vi "Test Publish QoS 0 Latency.vi"() -> ()   [LabVIEW 2013]
uses:
  <vilib>/LabVIEW Open Source Project/MQTT Control Packets/Control Packets/ControlPacket/Control Packet Type -- enum.ctl
  <vilib>/LabVIEW Open Source Project/MQTT Control Packets/Control Packets/ControlPacket/ControlPacket.lvclass
  <vilib>/LabVIEW Open Source Project/MQTT Control Packets/Control Packets/ControlPacket/QualityOfService -- enum.ctl
  <vilib>/LabVIEW Open Source Project/MQTT Control Packets/Control Packets/PUBLISH/PUBLISH.lvclass
  <vilib>/LabVIEW Open Source Project/MQTT Control Packets/Control Packets/ControlPacket/ControlPacket.lvclass/ControlPacket.ctl
  source/Client class/Client.lvclass
  <vilib>/LabVIEW Open Source Project/MQTT Connection/MQTT_Base/Base Class/MQTT_Base.lvclass
  <vilib>/LabVIEW Open Source Project/MQTT Control Packets/Control Packets/CONNACK/CONNACK.lvclass
  <vilib>/LabVIEW Open Source Project/Connection/Connection.TCP/Connection.TCP.lvclass
  <vilib>/LabVIEW Open Source Project/Connection/Connection/Connection.lvclass
panel:
  out "Raw Reception Latency (s)":dbl
  out "bytes received":i32
  out "Waveform Chart":cluster{dbl, dbl}(graph)
  out "# Bytes in payload":i32[](array[numeric])
  out "Disconnected by peer":bool
  out "# packets received":i32
  out "Raw Publication Latency (s)":dbl
  out "Topic":string[](array[string])
  out "Packet Type":T1[](array[typedef])
  out "server connected":bool
  out "listener error":errorcluster
  out "error out":errorcluster
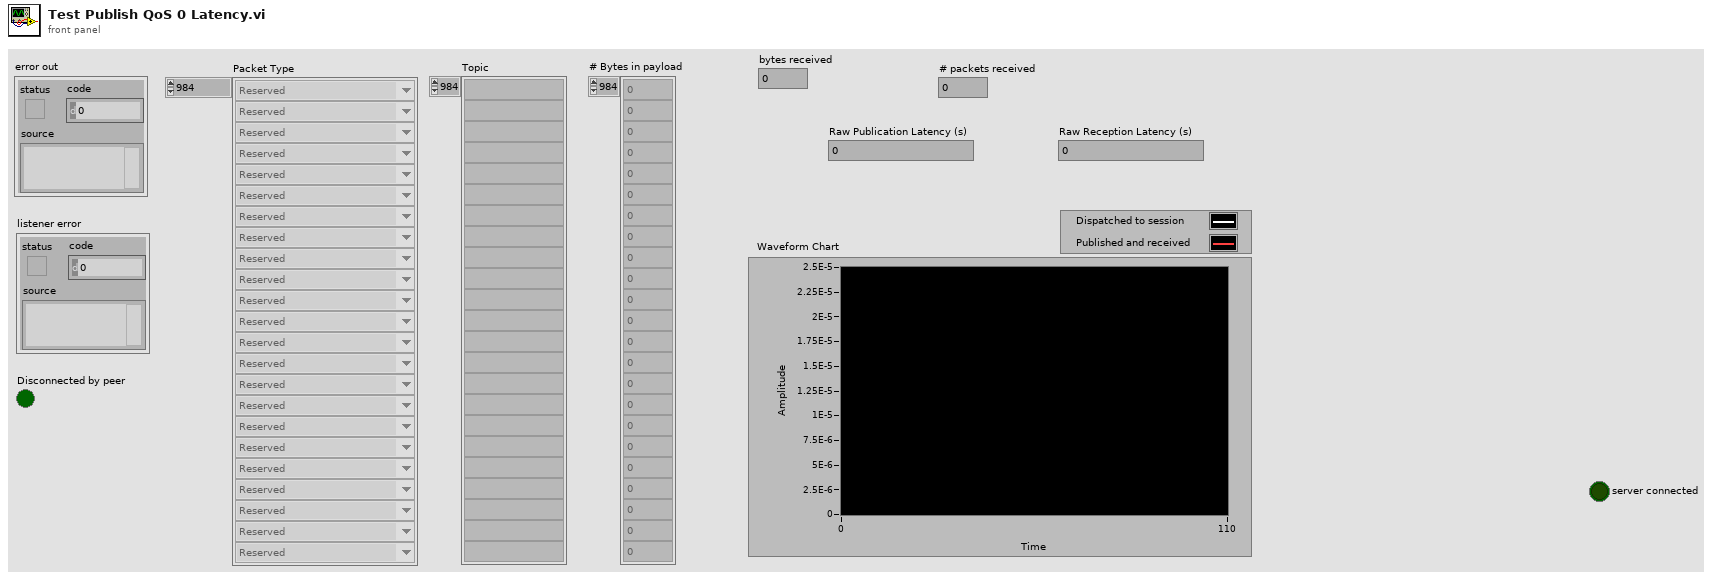
[diagram p1: front panel]
types:
  T1 = typedef "MQTT_Control_Packets.lvlib/ControlPacket.lvclass/Control Packet Type -- enum.ctl" = enum16{"Reserved", "CONNECT", "CONNACK", "PUBLISH", "PUBACK", "PUBREC", "PUBREL", "PUBCOMP", "SUBSCRIBE", "SUBACK", "UNSUBSCRIBE", "UNSUBACK", "PINGREQ", "PINGRESP", "DISCONNECT", "AUTH"}
  T2 = enum16{"Standard", "Buffered", "CRLF", "Immediate"}
  T3 = typedef "MQTT_Control_Packets.lvlib/ControlPacket.lvclass/QualityOfService -- enum.ctl" = enum16{"0 (At Most Once)", "1 (At Least Once)", "2 (Exactly Once)"}
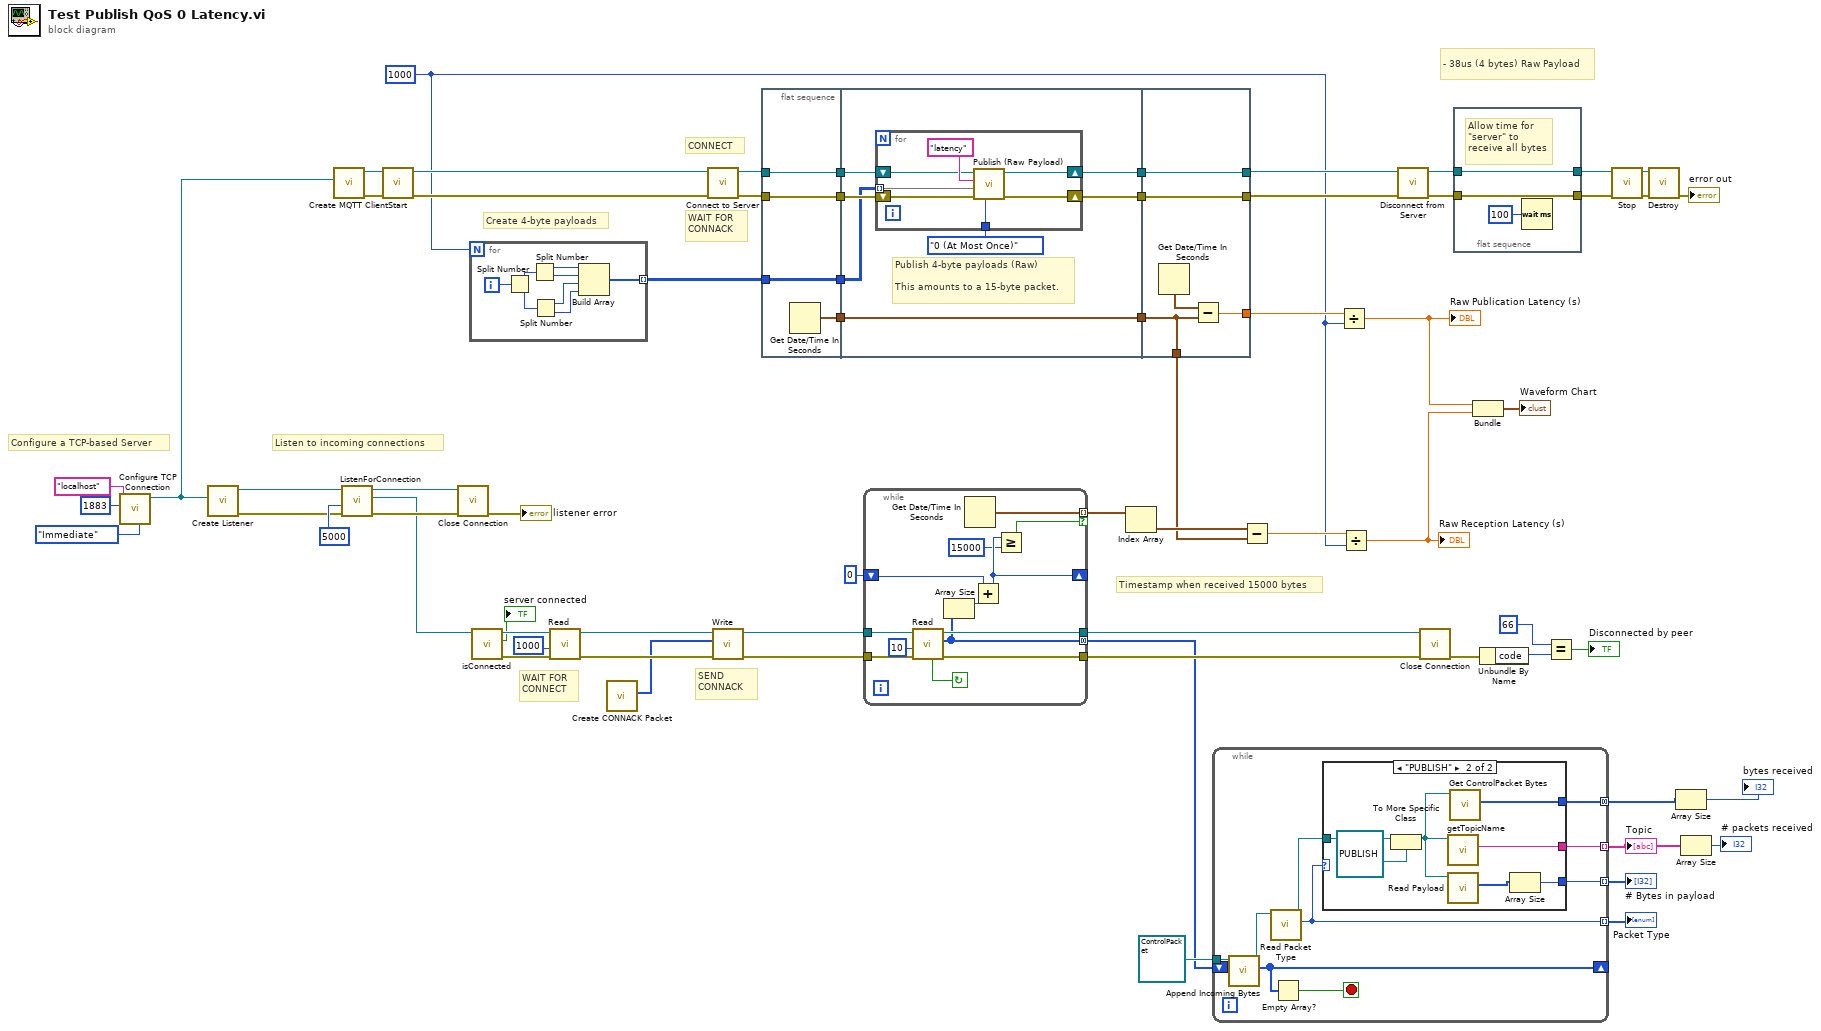
[diagram p0: block diagram]
diagram:
  w9 = 1000
  # "CONNECT"
  # "WAIT FOR\nCONNACK"
  # "Timestamp when received 15000 bytes"
  # "SEND \nCONNACK"
  # "WAIT FOR\nCONNECT"
  # "- 38us (4 bytes) Raw Payload"
  # "Create 4-byte payloads"
  # "Listen to incoming connections"
  # "Configure a TCP-based Server"
  n1 = call <vilib>:"Configure TCP Connection.vi"("Read Mode (Immediate)"=T2."Immediate", "remote port (80)"=u16 1883, "address (localhost)"="localhost") -> ("Connection.TCP"=w3:refnum<class "Connection.TCP.lvclass">)  [unwired: 7 in, 1 out]
  n2 = call <vilib>:"Create Listener.vi"("Connection Configuration"=w3) -> ("error out"=w2:errorcluster, "Listener"=w1:refnum<class "Connection.TCP.lvclass">)  [unwired: 9 in]
  n3 = call "Create MQTT Client.vi"("Connection Configuration"=w3) -> ("error out"=w66:errorcluster, "Client out"=w64:refnum<class "Client.lvclass">)  [unwired: 9 in]
  n4 = call <vilib>:"ListenForConnection.vi"("error in (no error)"=w2, "timeout (2000 ms)"=5000 ("bytes to read (100)"), "Listener"=w1) -> ("error out"=w59:errorcluster, "Connection"=w54:refnum<class "Connection.lvclass">, "Listener out"=w60:refnum<class "Connection.TCP.lvclass">)  [unwired: 5 in, 1 out]
  n5 = call <vilib>:"Start.vi"("error in (no error)"=w66, "MQTT_Base in"=w64) -> ("error out"=w65:errorcluster, "MQTT_Base out"=w63:refnum<class "Client.lvclass">)  [unwired: 7 in, 1 out]
  n6 = call <vilib>:"Close Connection.vi"("error in (no error)"=w59, "Connection in"=w60) -> ("error out"=→"listener error":errorcluster)  [unwired: 8 in, 1 out]
  n7 = for {
    N: w9 -> [_]
    tunnel: [w68] -> w44 mode=indexing
    i -> [w75]
    n8 = Split Number(x=w75) -> (hi(x)=w74:u16, lo(x)=w73:u16)
    n9 = Split Number(x=w74) -> (hi(x)=w72:u8, lo(x)=w71:u8)
    n10 = Split Number(x=w73) -> (hi(x)=w70:u8, lo(x)=w69:u8)
    n11 = Build Array(w72, w71, w70, w69) -> (w68:u8[])
  }
  n12 = call <vilib>:"isConnected.vi"("Connection in"=w54) -> ("error out"=w32:errorcluster, "connected"=→"server connected":bool, "Connection out"=w33:refnum<class "Connection.lvclass">)  [unwired: 8 in]
  n13 = call <vilib>:"Read.vi"("error in (no error)"=w32, "timeout (2000 ms)"=1000 ("bytes to read (100)"), "TCPConnection in"=w33) -> ("error out"=w34:errorcluster, "TCPConnection out"=w35:refnum<class "Connection.lvclass">)  [unwired: 4 in, 3 out]
  n14 = call <vilib>:"Create CONNACK Packet.vi"() -> ("Bytes Stream"=w30:u8[])  [unwired: 9 in, 2 out]
  n15 = call "Connect to Server.vi"("error in (no error)"=w65, "Client in"=w63) -> ("error out"=w53:errorcluster, "Client out"=w51:refnum<class "Client.lvclass">)  [unwired: 6 in, 2 out]
  n16 = call <vilib>:"Write.vi"("error in (no error)"=w34, "Bytes"=w30, "Connection in"=w35) -> ("error out"=w28:errorcluster, "Connection"=w29:refnum<class "Connection.lvclass">)  [unwired: 7 in]
  n17 = flat-sequence {
    tunnel: w51 -> [w78]
    tunnel: w53 -> [w79]
    tunnel: [w79] -> w49
    tunnel: [w78] -> w48
    tunnel: [w77] -> w45
    tunnel: w44 -> [w77]
    tunnel: [w76] -> w43
    tunnel: w49 -> [w86]
    tunnel: w48 -> [w84]
    tunnel: [w85] -> w47
    tunnel: [w83] -> w46
    tunnel: w45 -> [w82]
    tunnel: w43 -> [w80]
    tunnel: [w80] -> w42
    tunnel: [w97] -> w50
    tunnel: [w98] -> w52
    tunnel: w47 -> [w98]
    tunnel: w46 -> [w97]
    tunnel: w42 -> [w94]
    tunnel: [w95] -> w41
    tunnel: [w94] -> w5
    frame #0 {
      n18 = Get Date/Time In Seconds() -> (seconds since 1Jan1904=w76:timestamp)
    }
    frame #1 {
      # "Publish 4-byte payloads (Raw)\n\nThis amounts to a 15-byte packet."
      n19 = for {
        shift-right: [w91] -> w85
        shift-left: w86 -> [w90]
        shift-right: [w89] -> w83
        shift-left: w84 -> [w92]
        tunnel: w82 -> [w88] mode=indexing
        tunnel: QualityOfService_--_enum."0 (At Most Once)" ("QoS") -> [w87]
        n20 = call "Publish (Raw Payload).vi"("QoS"=w87, "error in (no error)"=w90, "Binary Payload"=w88, "Topic Name"="latency", "Client in"=w92) -> ("error out"=w91:errorcluster, "Client out"=w89:refnum<class "Client.lvclass">)  [unwired: 4 in, 1 out]
      }
    }
    frame #2 {
      n21 = Get Date/Time In Seconds() -> (seconds since 1Jan1904=w96:timestamp)
      n22 = Subtract(x=w96, y=w94) -> (x-y=w95:dbl)
    }
  }
  n23 = while {
    tunnel: w29 -> [w110]
    tunnel: w28 -> [w109]
    tunnel: [w108] -> w27
    tunnel: [w107] -> w26
    tunnel: [w105] -> w16 mode=concatenating
    shift-right: [w102] -> _
    shift-left: 0 ("size(s)") -> [w103]
    tunnel: [w100] -> w12 mode=indexing if=w99
    stop <- w106 continue-if-true
    n24 = call <vilib>:"Read.vi"("error in (no error)"=w109, "timeout (2000 ms)"=10 ("bytes to read (100)"), "TCPConnection in"=w110) -> ("error out"=w107:errorcluster, "Bytes"=w105:u8[], "TCPConnection out"=w108:refnum<class "Connection.lvclass">, "connected"=w106:bool)  [unwired: 4 in, 1 out]
    n25 = Array Size(array=w105) -> (size(s)=w104:i32)
    n26 = Get Date/Time In Seconds() -> (seconds since 1Jan1904=w100:timestamp)
    n27 = Add(x=w103, y=w104) -> (x+y=w102:i32)
    n28 = Greater Or Equal?(x=w102, y=15000) -> (x >= y?=w99:bool)
  }
  n29 = Index Array(array=w12) -> (element=w11:timestamp)  [unwired: 1 in]
  n30 = while {
    tunnel: refnum<class "ControlPacket.lvclass"> refnum ("Incomplete ControlPacket") -> [w120]
    shift-right: [w119] -> _
    shift-left: w16 -> [w121]
    tunnel: [w116] -> w24 mode=indexing
    tunnel: [w114] -> w23 mode=indexing
    tunnel: [w113] -> w17 mode=indexing
    tunnel: [w112] -> w15 mode=concatenating
    stop <- w118 stop-if-true
    n31 = call <vilib>:"Append Incoming Bytes.vi"("Incoming Packets"=w121, "Incomplete ControlPacket"=w120) -> ("Remaining Packets"=w119:u8[], "ControlPacket"=w117:refnum<class "ControlPacket.lvclass">)  [unwired: 6 in, 2 out]
    n32 = call <vilib>:"Read Packet Type.vi"("ControlPacket in"=w117) -> ("Control Packet Type"=w116:T1, "ControlPacket out"=w115:refnum<class "ControlPacket.lvclass">)  [unwired: 9 in]
    n33 = Empty Array?(array=w119) -> (empty?=w118:bool)
    n34 = case shown="\"PUBLISH\"" w116 {
      tunnel: w115 -> [_ w128]
      tunnel: [_ w126] -> w114
      tunnel: [_ w124] -> w113
      tunnel: [_ w122] -> w112
      frame Default {
      }
      frame "PUBLISH" {
        n35 = To More Specific Class(target class=refnum<class "PUBLISH.lvclass"> refnum ("PUBLISH in"), reference=w128) -> (specific class reference=w123:refnum<class "PUBLISH.lvclass">)  [unwired: 1 in, 1 out]
        n36 = call <vilib>:"getTopicName.vi"("PUBLISH in"=w123) -> ("Topic"=w126:string)  [unwired: 8 in, 2 out]
        n37 = call <vilib>:"Read Payload.vi"("ControlPacket in"=w123) -> ("Payload"=w125:u8[])  [unwired: 9 in, 1 out]
        n38 = call <vilib>:"Get ControlPacket Bytes.vi"("ControlPacket"=w123) -> ("Bytes Stream"=w122:u8[])  [unwired: 7 in, 3 out]
        n39 = Array Size(array=w125) -> (size(s)=w124:i32)
      }
    }
  }
  "Packet Type" <- w24
  "Topic" <- w23
  "# Bytes in payload" <- w17
  n40 = Subtract(x=w11, y=w5) -> (x-y=w10:dbl)
  n41 = Divide(x=w41, y=w9) -> (x/y=w7:dbl)
  "Raw Publication Latency (s)" <- w7
  n42 = Divide(x=w10, y=w9) -> (x/y=w8:dbl)
  "Raw Reception Latency (s)" <- w8
  n43 = call "Disconnect from Server.vi"("error in (no error)"=w52, "Client in"=w50) -> ("error out"=w38:errorcluster, "Client out"=w40:refnum<class "Client.lvclass">)  [unwired: 7 in, 1 out]
  n44 = call <vilib>:"Close Connection.vi"("error in (no error)"=w26, "Connection in"=w27) -> ("error out"=w21:errorcluster)  [unwired: 8 in, 1 out]
  n45 = flat-sequence {
    tunnel: w40 -> [w131]
    tunnel: [w131] -> w39
    tunnel: w38 -> [w130]
    tunnel: [w130] -> w37
    frame #0 {
      # "Allow time for\n\"server\" to\nreceive all bytes"
      n46 = Wait (ms)(milliseconds to wait=u32 100) -> ()  [unwired: 1 out]
    }
  }
  n47 = Bundle(w7, w8) -> (→"Waveform Chart":cluster{dbl, dbl})  [unwired: 1 in]
  n48 = Unbundle By Name(w21) -> ("code"=w20:i32)
  n49 = Equal?(x=66, y=w20) -> (x = y?=→"Disconnected by peer":bool)
  n50 = call <vilib>:"Stop.vi"("error in (no error)"=w37, "MQTT_Base in"=w39) -> ("error out"=w61:errorcluster, "MQTT_Base out"=w62:refnum<class "Client.lvclass">)  [unwired: 7 in, 1 out]
  n51 = call <vilib>:"Destroy.vi"("error in (no error)"=w61, "MQTT_Base in"=w62) -> ("error out"=→"error out":errorcluster)  [unwired: 8 in, 1 out]
  n52 = Array Size(array=w15) -> (size(s)=→"bytes received":i32)
  n53 = Array Size(array=w23) -> (size(s)=→"# packets received":i32)
